vi "Verify Adaptive Agitate Profile ID and time.vi"(0 "GEA2 Reference In":refnum<k24>, 5 "ECT Data In":T1, 11 "Error In":errorcluster) -> (2 "Motor Profile ID Pass/Fail":bool, 3 "Expected SSD":string, 4 "GEA2 Reference Out":refnum<k24>, 6 "Actual ECT After Agitate (sec)":u16, 8 "Expected ECT After Agitate (sec)":u16, 10 "ECT After Agitate Pass/Fail":bool, 13 "Agi Profile Report":string, 14 "Report Text":string, 15 "Error Out":errorcluster)   [LabVIEW 2016, in "TLMB.lvlib"]
doc: "This vi can be used to read ERD every 1 sec for user selected repeat counts."
uses:
  Projects/TLMB.lvlib
  Q:/Common/DLLs/GEA3/GeaCommunication.dll
  Common/DLLs/GEA3/GeaCommunication.dll
  Controls/ECT.ctl
  Common/LabVIEW GEA2 Toolkit/LabVIEW_GEA2_Toolkit.lvlibp/type defs/Source_Destination.ctl
  Common/LabVIEW GEA2 Toolkit/LabVIEW_GEA2_Toolkit.lvlibp/type defs/ERD Read Data In.ctl
  Common/LabVIEW GEA2 Toolkit/LabVIEW_GEA2_Toolkit.lvlibp/type defs/Data Type.ctl
  Common/LabVIEW GEA2 Toolkit/LabVIEW_GEA2_Toolkit.lvlibp
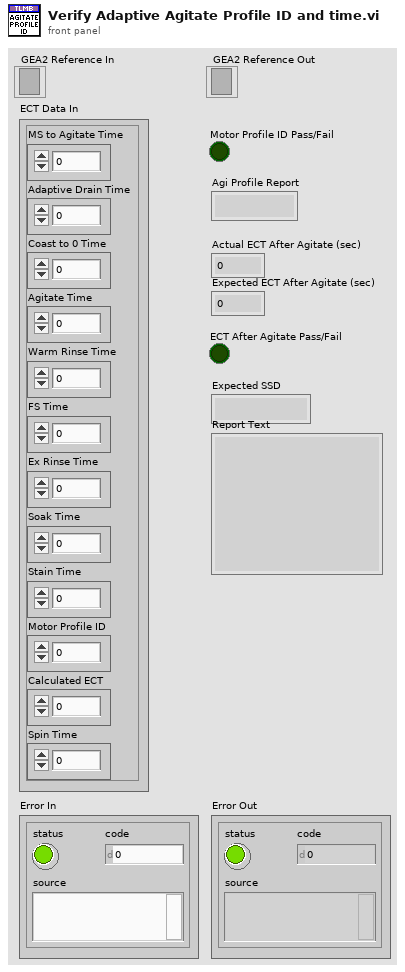
[diagram p1: front panel]
types:
  T1 = typedef "TLMB.lvlib/ECT.ctl" = cluster{"MS to Agitate Time":u16, "Adaptive Drain Time":u16, "Coast to 0 Time":u16, "Agitate Time":u16, "Warm Rinse Time":u16, "FS Time":u16, "Ex Rinse Time":u16, "Soak Time":u16, "Stain Time":u16, "Motor Profile ID":u16, "Calculated ECT":u16, "Spin Time":u16}
  T2 = typedef "LabVIEW_GEA2_Toolkit.lvlibp/Source_Destination.ctl" = cluster{"Source":u8, "Destination":u8}
  T3 = typedef "LabVIEW_GEA2_Toolkit.lvlibp/ERD Read Data In.ctl" = cluster{"ERD Number":u16, "Data Type":T4}
  T4 = typedef "LabVIEW_GEA2_Toolkit.lvlibp/Data Type.ctl" = enum16{"string", "boolean", "uint8_t", "uint16_t", "uint32_t", "uint64_t", "int8_t", "int16_t", "int32_t", "int64_t"}
  T5 = enum16{"EQ (==)", "NE (!=)", "GT (>)", "LT (<)", "GE (>=)", "LE (<=)", "GTLT(> <)", "GELE (>= <=)", "GELT (>= <)", "GTLE (> <=)", "LTGT (< >)", "LEGE (<= >=)", "LEGT (<= >)", "LTGE (< >=)", "No Comparison"}
  T6 = typedef "LabVIEW_GEA2_Toolkit.lvlibp/ERD Read Data Out.ctl" = cluster{"ERD Number":u16, "Data":string}
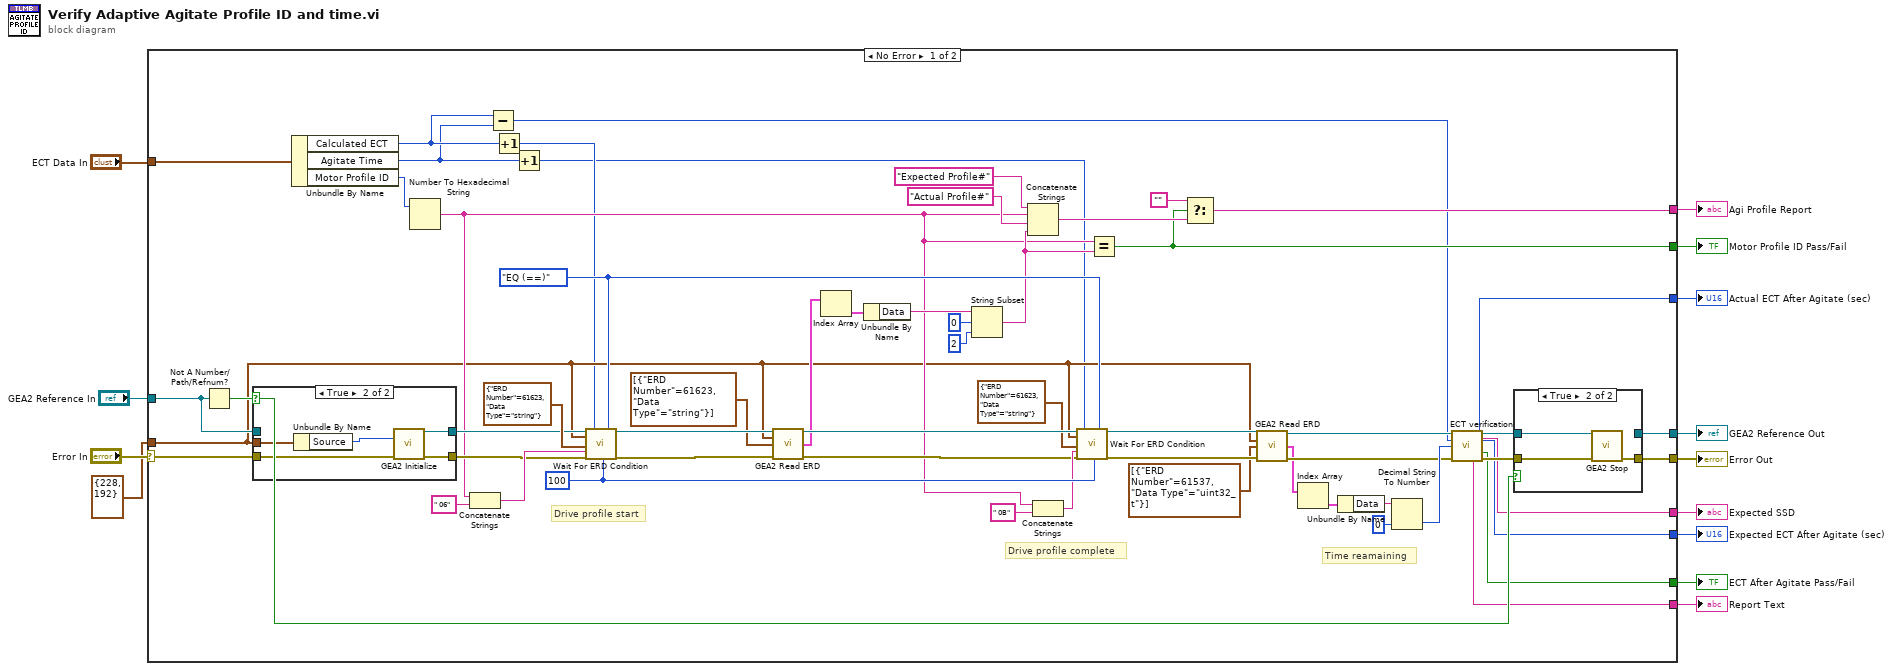
[diagram p0: block diagram]
diagram:
  n1 = case shown="No Error" "Error In" {
    selector: "Error In" -> [w70 w84]
    tunnel: T2 {"Source"=228, "Destination"=192} ("GEA Inputs") -> [w26 _]
    tunnel: "GEA2 Reference In" -> [w71 w85]
    tunnel: [w67 w85] -> w11
    tunnel: [w69 w84] -> w10
    tunnel: "ECT Data In" -> [w14 _]
    tunnel: [w64 _] -> w9
    tunnel: [w63 _] -> w8
    tunnel: [w53 _] -> w5
    tunnel: [w52 _] -> w4
    tunnel: [w51 _] -> w3
    tunnel: [w50 _] -> w6
    tunnel: [w32 _] -> w2
    frame No Error {
      w58 = u32 100 ("Loop Rate (ms)")
      w57 = T5."EQ (==)" ("Comparison")
      # "Time reamaining"
      # "Drive profile complete"
      # "Drive profile start"
      n2 = Not A Number/Path/Refnum?(number/path/refnum=w71) -> (NaN/Path/Refnum?=w68:bool)
      n3 = case shown="True" w68 {
        tunnel: w70 -> [w78 w83]
        tunnel: [w78 w82] -> w48
        tunnel: [w77 w81] -> w49
        tunnel: w26 -> [_ w79]
        tunnel: w71 -> [w77 _]
        frame False {
        }
        frame True {
          n4 = Unbundle By Name(w79) -> ("Source"=w80:u8)
          n5 = call "GEA2 Initialize.vi"("Source Address"=w80, "error in"=w83) -> ("GEA2 Reference Out"=w81:refnum<k24>, "error out"=w82:errorcluster)  [unwired: 11 in, 1 out]
        }
      }
      n6 = Unbundle By Name(w14) -> ("Calculated ECT"=w21:u16, "Agitate Time"=w18:u16, "Motor Profile ID"=w22:u16)
      n7 = Number To Hexadecimal String(2:w22) -> (0:w34:string)  [unwired: 1 in]
      n8 = Concatenate Strings(w34, " 06" ("string")) -> (w60:string)
      n9 = Subtract(x=w21, y=w18) -> (x-y=w23:u16)
      n10 = Increment(x=w21) -> (x+1=w20:u16)
      n11 = Increment(x=w18) -> (x+1=w19:u16)
      n12 = call "Wait For ERD Condition.vi"("GEA2 Reference In"=w49, "GEA Inputs"=w26, "ERD Read Data"=T3 {"ERD Number"=61623, "Data Type"=enum."string"}, "Expected Low"=w60, "Error In"=w48, "Timeout (s)"=w20, "Loop Rate (ms)"=w58, "Comparison"=w57) -> ("GEA2 Reference Out"=w43:refnum<k24>, "Error Out"=w42:errorcluster)  [unwired: 7 in, 3 out]
      n13 = call "GEA2 Read ERD.vi"("GEA2 Reference In"=w43, "GEA Inputs"=w26, "Read ERD List"=T3[] [{"ERD Number"=61623, "Data Type"=enum."string"}], "Error In"=w42) -> ("GEA2 Reference Out"=w40:refnum<k24>, "ERD Data Out"=w39:T6[], "Error Out"=w41:errorcluster)  [unwired: 8 in, 1 out]
      n14 = Index Array(array=w39) -> (element=w46:T6)  [unwired: 1 in]
      n15 = Unbundle By Name(w46) -> ("Data"=w47:string)
      n16 = String Subset(string=w47, offset (0)=0, length (rest)=2 ("length (rest)")) -> (substring=w35:string)
      n17 = Concatenate Strings("Expected Profile#", w34, "Actual Profile#", w35) -> (w66:string)
      n18 = Concatenate Strings(w34, " 0B" ("string")) -> (w56:string)
      n19 = call "Wait For ERD Condition.vi"("GEA2 Reference In"=w40, "GEA Inputs"=w26, "ERD Read Data"=T3 {"ERD Number"=61623, "Data Type"=enum."string"}, "Expected Low"=w56, "Error In"=w41, "Timeout (s)"=w19, "Loop Rate (ms)"=w58, "Comparison"=w57) -> ("GEA2 Reference Out"=w30:refnum<k24>, "Error Out"=w28:errorcluster)  [unwired: 7 in, 3 out]
      n20 = Equal?(x=w34, y=w35) -> (x = y?=w64:bool)
      n21 = Select(t="", s=w64, f=w66) -> (s? t:f=w63:string)
      n22 = call "GEA2 Read ERD.vi"("GEA2 Reference In"=w30, "GEA Inputs"=w26, "Read ERD List"=T3[] [{"ERD Number"=61537, "Data Type"=enum."uint32_t"}], "Error In"=w28) -> ("GEA2 Reference Out"=w29:refnum<k24>, "ERD Data Out"=w24:T6[], "Error Out"=w27:errorcluster)  [unwired: 8 in, 1 out]
      n23 = Index Array(array=w24) -> (element=w38:T6)  [unwired: 1 in]
      n24 = Unbundle By Name(w38) -> ("Data"=w37:string)
      n25 = Decimal String To Number(string=w37, default (0L)=u16 0 ("Expected ECT After Agitate (sec)")) -> (number=w31:u16)  [unwired: 1 in, 1 out]
      n26 = call "ECT verification.vi"(".NET Refnum in"=w29, "Cal ECT (sec)"=w23, "Time remaining (sec)"=w31, "error in"=w27) -> ("Expected SSD"=w52:string, ".NET Refnum out"=w55:refnum<k24>, "Expected ECT (sec)"=w53:u16, "Actual ECT (sec)"=w50:u16, "ECT Pass/Fail"=w32:bool, "Report Text"=w51:string, "error out"=w54:errorcluster)  [unwired: 5 in]
      n27 = case shown="True" w68 {
        tunnel: [w73 w76] -> w69
        tunnel: w55 -> [w72 w75]
        tunnel: w54 -> [w73 w74]
        tunnel: [w72 _] -> w67
        frame False {
        }
        frame True {
          n28 = call "GEA2 Stop.vi"("GEA2 Reference In"=w75, "Error In"=w74) -> ("Error Out"=w76:errorcluster)  [unwired: 13 in]
        }
      }
    }
    frame Error {
    }
  }
  "GEA2 Reference Out" <- w11
  "Error Out" <- w10
  "Motor Profile ID Pass/Fail" <- w9
  "Agi Profile Report" <- w8
  "Actual ECT After Agitate (sec)" <- w6
  "Expected ECT After Agitate (sec)" <- w5
  "Expected SSD" <- w4
  "Report Text" <- w3
  "ECT After Agitate Pass/Fail" <- w2
